vi "LET Output v1.vi"() -> ()   [LabVIEW 2010]
doc: "Cont(inuous) Acq(uire) & Chart (hw timed) demonstrates the hardware timed, non-buffered technique of data acquisition. The scan clock on the board controls acquisition timing. Acquired scans are read directly from the device's FIFO using AI Single Scan. \n\nThe acquisition is configured with no buffer, and the on-board scan clock started at the selected scan rate. In the first loop iteration, the newest (most recent) scan is read from the FIFO. In each subsequent loop iteration AI Single Scan is called to read the oldest scan from the FIFO. Then if a scan is missed because the acquisition does not keep up, an error message will be displayed, and the acquisition stopped. Each scan is plotted on the chart after it is read. \n\nA common reason to use non-buffered acquisition is that some kind of processing needs to be done for each data point. You will probably want to add more functions to the diagram to customize this VI for your application. The acquisition rate you can achieve depends on how much processing and display the VI must do. This VI calls a subVI named My Single-Scan Processing. Add whatever processing you need to this subVI, or replace it with one of your own. The data processing subVI also demonstrates how to use error clusters in your own subVIs, so they can be included in the error data flow chain.\n\nBefore running this VI, set the values of the controls on the front panel. Select Show Help Window from the Help menu to see a description of each control. If the values you select for all the controls are values you will usually use, select Make Current Values Default from the Operate menu and save the VI. Or, you may save individual control's default values by popping up on the control, selecting Data Operations, then selecting Make Current Value Default, and saving the VI."
uses:
  <instrlib>/agilent_b2900_series/Agilent B2900 Series/Public/Configure/Measurement/Configure Measurement (Current).vi
  <instrlib>/agilent_b2900_series/Agilent B2900 Series/Public/Configure/Measurement/Configure Measurement (Voltage).vi
  <vilib>/Utility/file.llb/Write To Spreadsheet File (DBL).vi
  <instrlib>/agilent_b2900_series/Agilent B2900 Series/Agilent B2900 Series.lvlib
panel:
  out "Igs array 2":dbl[][](array[numeric])
  out "Vgs array 2":dbl[][](array[numeric])
  out "Vds array 2":dbl[][](array[numeric])
  out "Corrected PD current array 2":dbl[][](array[numeric])
  out "Ids array 2":dbl[][](array[numeric])
  out "corrected PD current array":dbl[](array[numeric])
  out "Vds array":dbl[](array[numeric])
  out "Ids array":dbl[](array[numeric])
  out "Vgs array":dbl[](array[numeric])
  out "Igs array":dbl[](array[numeric])
  in  "Tab Control":T1(tab)
  in  "keithley address":string="GPIB0::20::INSTR"
  in  "agilent address":refnum<visa-resource-name>="GPIB0::23::INSTR"
  in  "Initial Vds (V)\n(100 scans/sec)":sgl caption="Initial Vds (V)" format="%.2f"
  in  "Vds step (V)":sgl=1.0 format="%.2f"
  in  "Vds delay time":sgl=10.0 caption="Vds delay time (ms)" format="%.2f"
  in  "Vds delay after first value (ms)":sgl=10.0 format="%.2f"
  in  "Final Vds(V)":sgl=60.0 format="%.2f"
  in  "light emission ON/OFF":bool=TRUE
  in  "Vgs step (V)":sgl=20.0 format="%.2f"
  in  "Final Vgs (V)":sgl=60.0 format="%.2f"
  in  "Initial Vgs (V)":sgl format="%.2f"
  in  "Vgs hold time (ms)":i32=10
  in  "Compliance Voltage (channel 2)":dbl=60.0
  in  "Compliance Current (channel 1)":dbl=0.001
  in  "Compliance Voltage (channel 1)":dbl=60.0
  in  "Compliance Current (channel 2)":dbl=0.0001
  in  "keithley compliance limit":dbl(ring)=0.025 items=["25uA"=2.5e-05, "250uA"=0.00025, "2.5mA"=0.0025, "25mA"=0.025]
  in  "Loop":bool=TRUE
  out "Current Scan":cluster{dbl[], dbl[]}(graph)
  out "Applied Vds":sgl caption="current VDS (V)" format="%.2f"
  out "Applied Vgs":sgl caption="current VDS (V)" format="%.2f"
  out "Measured Ids":dbl format="%.2e"
  out "Measured Vds":dbl
  out "corrected PD current":dbl format="%^.2e"
  out "dark PD current (A)":dbl format="%^.2e"
  out "PD current":dbl format="%^.2e"
  out "Measured Igs":dbl
  out "Measured Vgs":dbl
  out "channel 2 status":bool
  out "channel 1 status":bool
  out "Current Scan 2":cluster{dbl[], dbl[]}(graph) caption="Current Scan"
  out "half  points":sgl
  out "Vds points":sgl
  out "Vgs points":sgl
  out "?":cluster{dbl[], dbl[]}[](graph)
  out "?":cluster{dbl[], dbl[]}[](graph)
  in  "error in keithley":errorcluster
  out "keithley address out":refnum<k15>
  out "error out keithley":errorcluster
  out "error out agilent":errorcluster
  out "Agilent address out":refnum<visa-resource-name>
  # "FET output v1"
  # "Drain-Source Setting"
  # "Gate Setting"
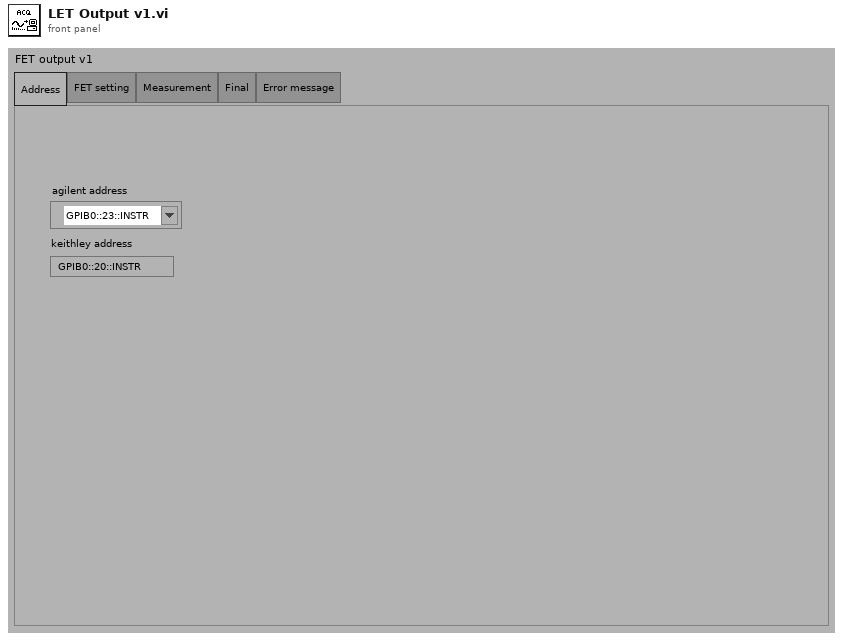
[diagram p1: front panel]
types:
  T1 = enum32{"Address", "FET setting", "Measurement", "Final", "Error message"}
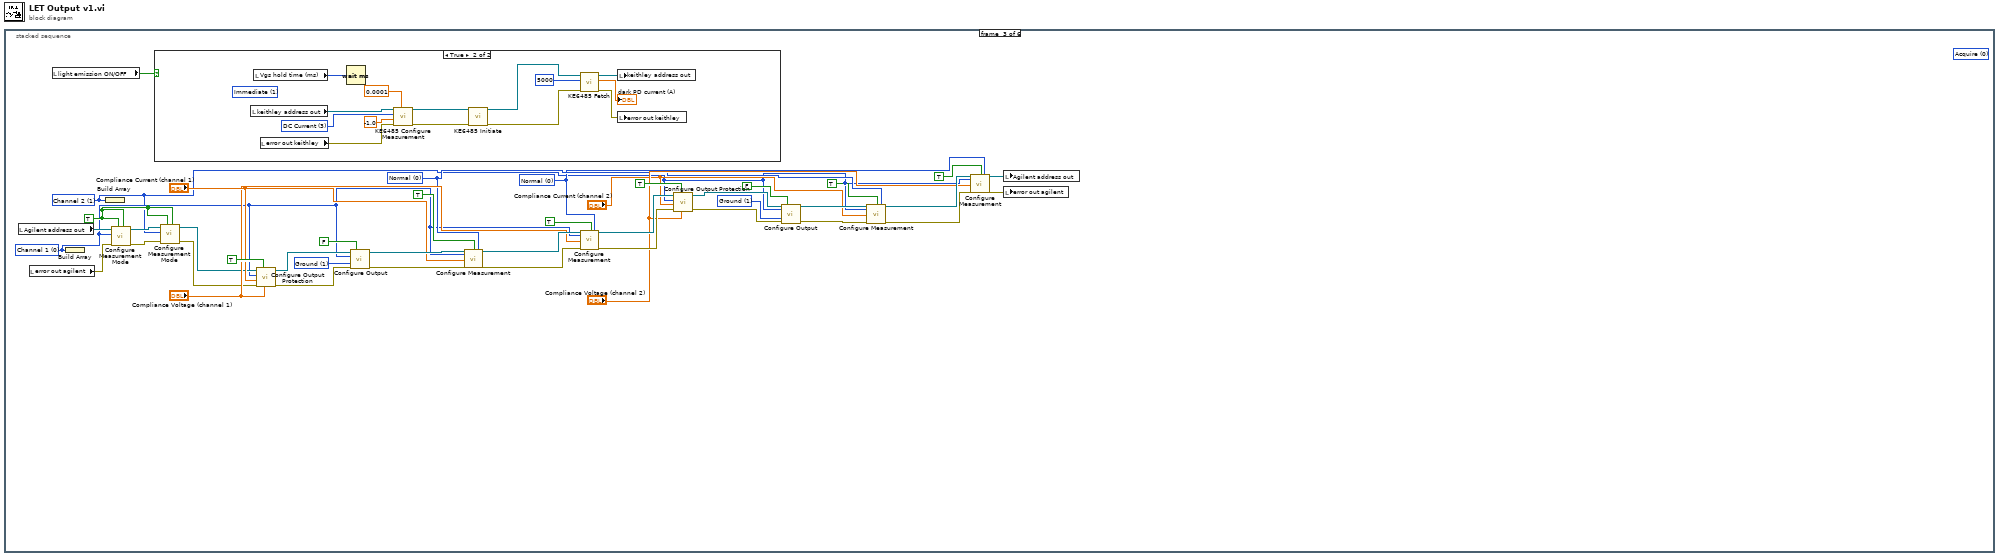
[diagram p0: block diagram]
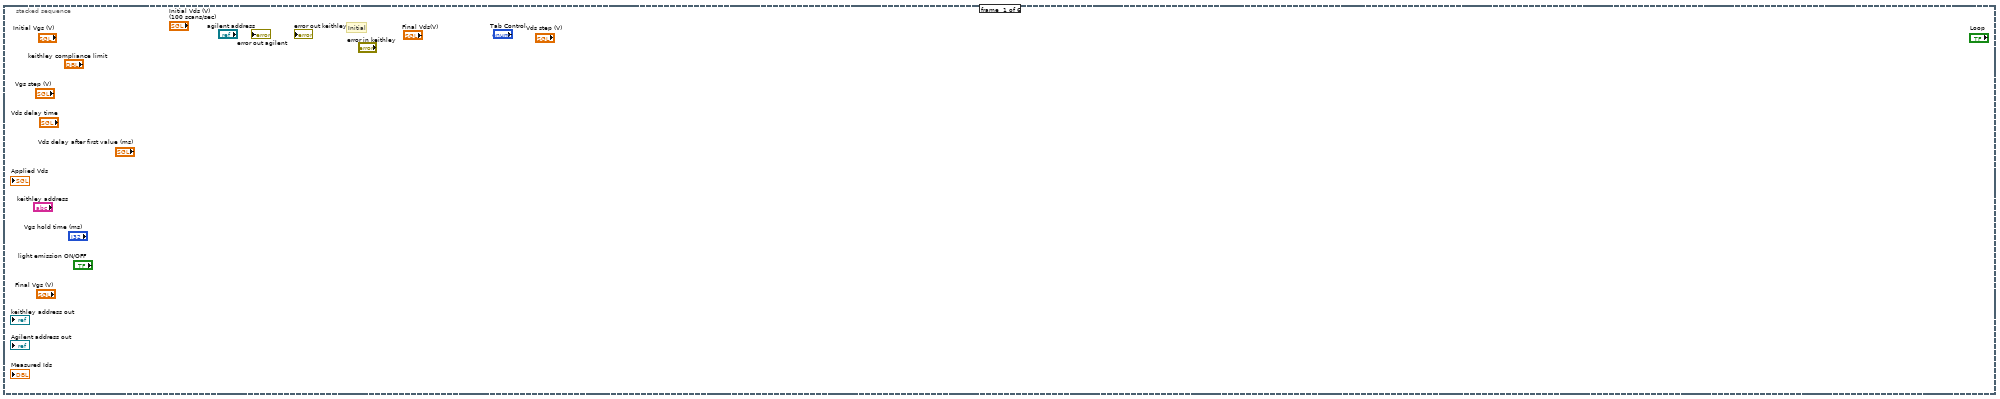
[diagram p2: hidden frame]
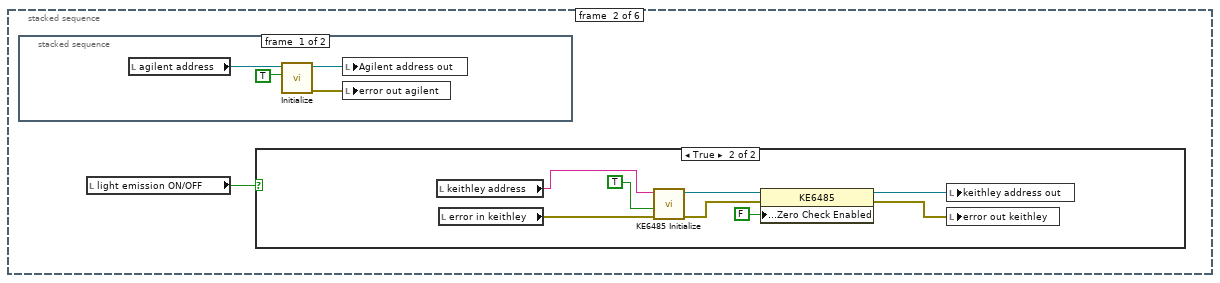
[diagram p3: hidden frame]
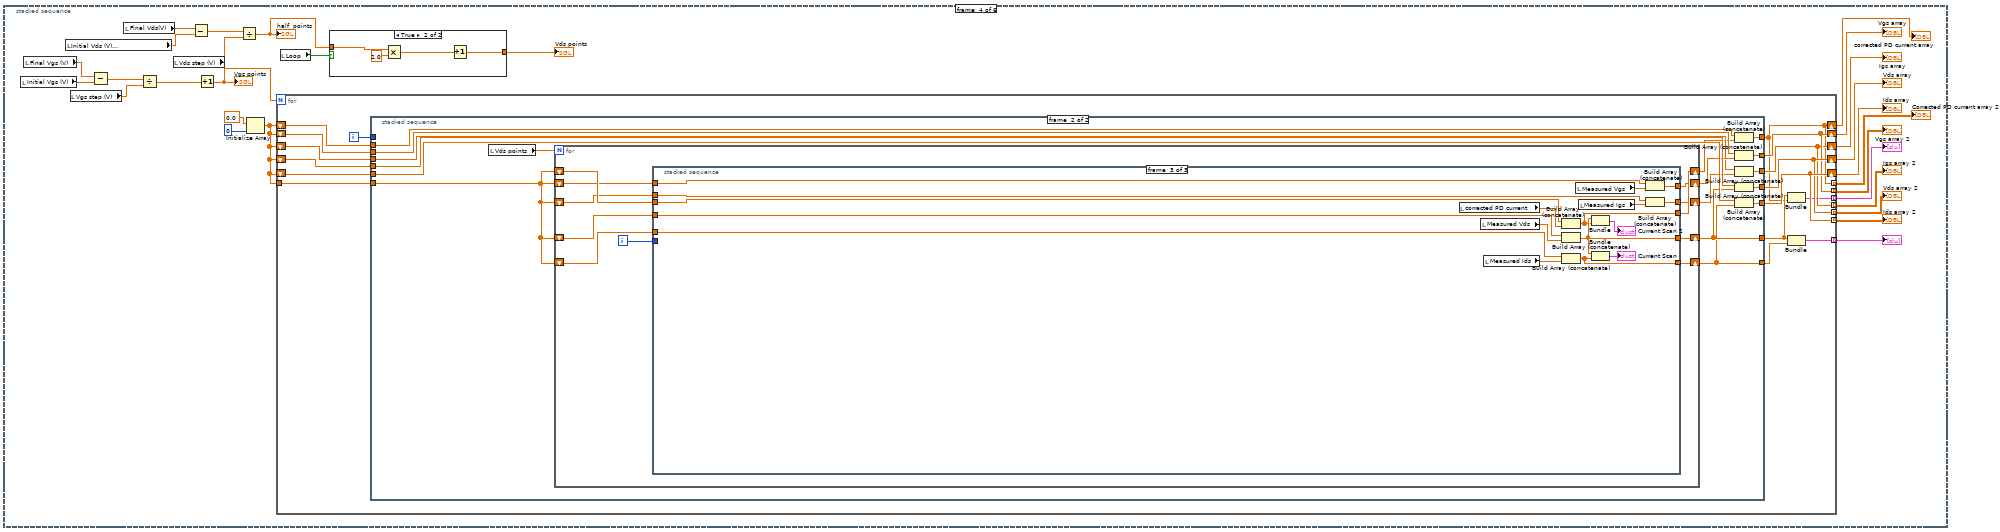
[diagram p7: hidden frame]
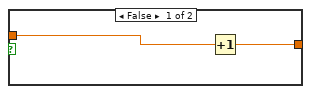
[diagram p8: hidden frame]
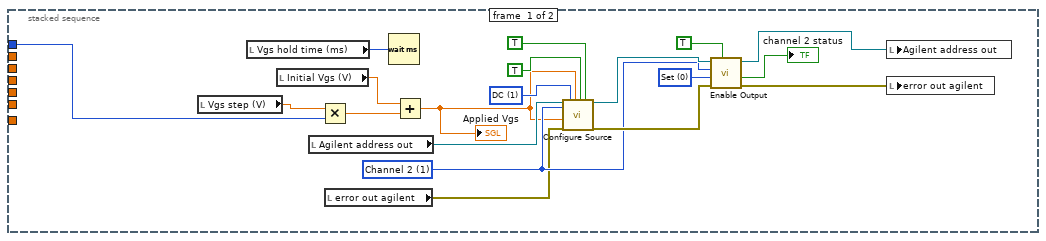
[diagram p9: hidden frame]
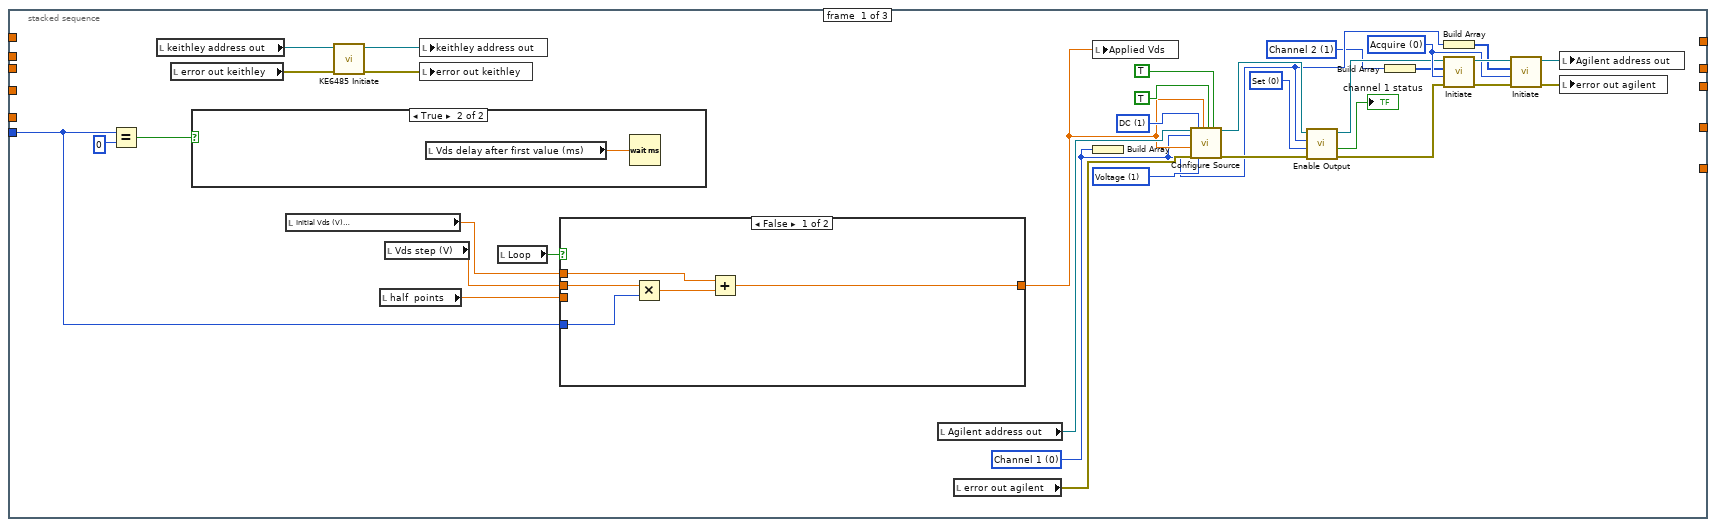
[diagram p10: hidden frame]
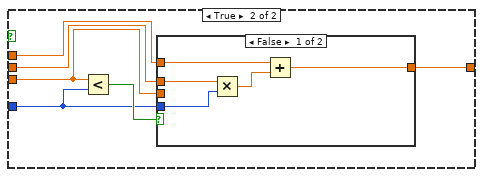
[diagram p11: hidden frame]
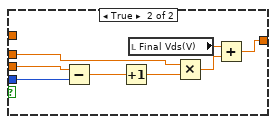
[diagram p12: hidden frame]
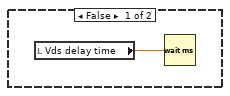
[diagram p13: hidden frame]
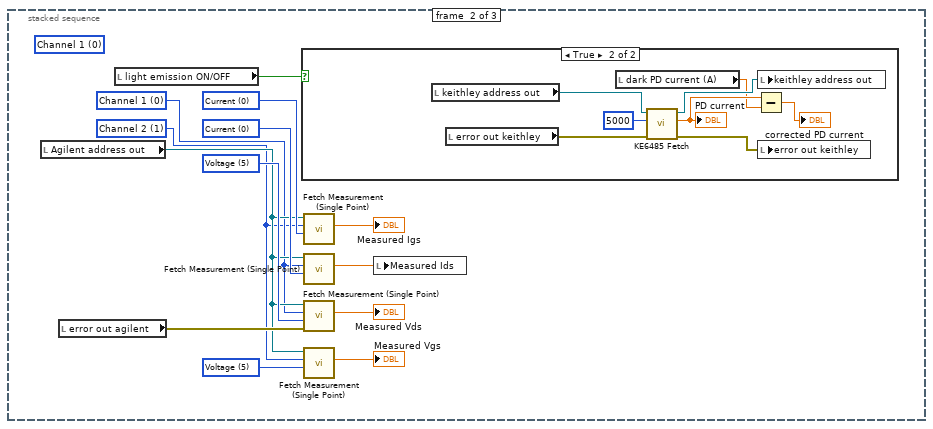
[diagram p14: hidden frame]
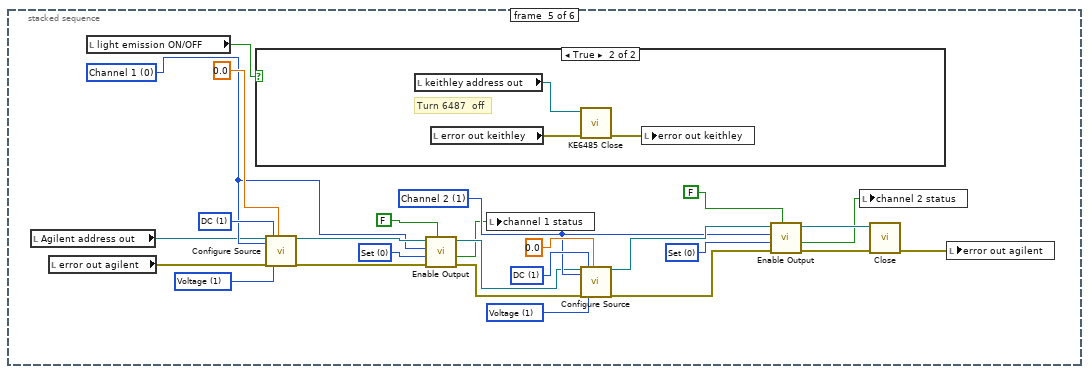
[diagram p16: hidden frame]
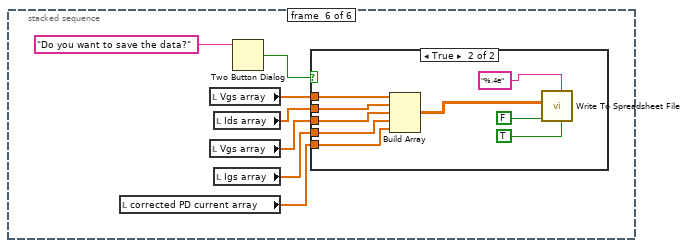
[diagram p18: hidden frame]
diagram:
  n1 = stacked-sequence {
    frame #0 {
      # "Initial"
    }
    frame #1 {
      n2 = stacked-sequence {
        frame #0 {
          n3 = local read "agilent address"() -> (w2:refnum<visa-resource-name>)
          n4 = call <instrlib>:"Initialize.vi"("ID Query (True)"=TRUE, "VISA resource name"=w2) -> ("error out"=w3:errorcluster, "VISA resource name out"=w4:refnum<visa-resource-name>)  [unwired: 8 in]
          n5 = local write "Agilent address out"(w4) -> ()
          n6 = local write "error out agilent"(w3) -> ()
        }
        frame #1 {
        }
      }
      n7 = local read "light emission ON/OFF"() -> (w1:bool)
      n8 = case shown="True" w1 {
        frame False {
        }
        frame True {
          n9 = local read "keithley address"() -> (w12:string)
          n10 = local read "error in keithley"() -> (w13:errorcluster)
          n11 = call <instrlib>:"KE6485 Initialize.vi"("error in (no error)"=w13, "reset device"=TRUE, "resource name"=w12) -> ("error out"=w10:errorcluster, "instrument handle out"=w9:refnum<k15>)  [unwired: 1 in, 6 out]
          n12 = property class="KE6485"(reference=w9, error in=w10, "System Settings:Zero Check Enabled"=FALSE) -> (reference out=w8:refnum<k15>, error out=w7:errorcluster)
          n13 = local write "keithley address out"(w8) -> ()
          n14 = local write "error out keithley"(w7) -> ()
        }
      }
    }
    frame #2 {
      (unwired) 0 items=["Acquire", "Transient", "Both"] ("Device Action (2: Both)")
      w24 = TRUE ("Enable Voltage Measurement (T: Enable)")
      w38 = 1 items=["Float", "Ground"] ("Low Terminal State (1: Ground)")
      w16 = 1 items=["Channel 1", "Channel 2"] ("Channel (0: Channel 1)")
      w26 = 0 items=["Normal", "Resolution", "Speed"] ("Current Auto Range Mode (0: Normal)")
      w48 = 1 items=["Float", "Ground"] ("Low Terminal State (1: Ground)")
      w17 = 0 items=["Channel 1", "Channel 2"] ("Channel (0: Channel 1)")
      w25 = 0 items=["Normal", "Resolution", "Speed"] ("Voltage Auto Range Mode (0: Normal)")
      n15 = local read "Agilent address out"() -> (w19:refnum<visa-resource-name>)
      n16 = local read "error out agilent"() -> (w21:errorcluster)
      n17 = local read "light emission ON/OFF"() -> (w55:bool)
      n18 = Build Array(w17) -> ()  [unwired: 1 out]
      n19 = Build Array(w16) -> ()  [unwired: 1 out]
      n20 = call <instrlib>:"Configure Measurement Mode.vi"("Enable Current Measurement (T: Enable)"=w24, "Enable Voltage Measurement (T: Enable)"=w24, "error in (no error)"=w21, "Channel (0: Channel 1)"=w17, "VISA resource name"=w19) -> ("error out"=w22:errorcluster, "VISA resource name out"=w23:refnum<visa-resource-name>)  [unwired: 5 in]
      n21 = case shown="True" w55 {
        frame False {
        }
        frame True {
          (unwired) 1 items=["Immediate"=1, "Interval"=10, "Trigger Link 1"=1001, "Trigger Link 2"=1002, "Trigger Link 3"=1003, "Trigger Link 4"=1004, "Trigger Link 5"=1005, "Trigger Link 6"=1006] ("sample trigger")
          w67 = 3 items=["DC Volts"=1, "DC Current"=3, "2 Wire Resistance"=5, "Charge"=1004] ("measurement function")
          n22 = local read "keithley address out"() -> (w62:refnum<k15>)
          n23 = local read "Vgs hold time (ms)"() -> (w69:i32)
          n24 = local read "error out keithley"() -> (w61:errorcluster)
          n25 = Wait (ms)(milliseconds to wait=w69) -> ()  [unwired: 1 out]
          n26 = call <instrlib>:"KE6485 Configure Measurement.vi"("resolution (absolute)"=0.0001, "error in (no error)"=w61, "range"=-1.0, "measurement function"=w67, "instrument handle"=w62) -> ("error out"=w58:errorcluster, "instrument handle out"=w60:refnum<k15>)  [unwired: 5 in]
          n27 = call <instrlib>:"KE6485 Initiate.vi"("error in (no error)"=w58, "instrument handle"=w60) -> ("error out"=w57:errorcluster, "instrument handle out"=w59:refnum<k15>)  [unwired: 8 in]
          n28 = call <instrlib>:"KE6485 Fetch.vi"("error in (no error)"=w57, "maximum time (ms)"=5000, "instrument handle"=w59) -> ("error out"=w64:errorcluster, "reading"=→"dark PD current (A)":dbl, "instrument handle out"=w63:refnum<k15>)  [unwired: 6 in]
          n29 = local write "keithley address out"(w63) -> ()
          n30 = local write "error out keithley"(w64) -> ()
        }
      }
      n31 = call <instrlib>:"Configure Measurement Mode.vi"("Enable Current Measurement (T: Enable)"=w24, "Enable Voltage Measurement (T: Enable)"=w24, "error in (no error)"=w22, "Channel (0: Channel 1)"=w16, "VISA resource name"=w23) -> ("error out"=w20:errorcluster, "VISA resource name out"=w18:refnum<visa-resource-name>)  [unwired: 5 in]
      n32 = call <instrlib>:"Configure Output Protection.vi"("Compliance Voltage (2 V)"="Compliance Voltage (channel 1)", "Enable Output Protection (T: Enable)"=TRUE, "error in (no error)"=w20, "Compliance Current (0.0001 A)"="Compliance Current (channel 1)", "Channel (0: Channel 1)"=w17, "VISA resource name"=w18) -> ("error out"=w50:errorcluster, "VISA resource name out"=w49:refnum<visa-resource-name>)  [unwired: 4 in]
      n33 = call <instrlib>:"Configure Output.vi"("VISA resource name"=w49, "Auto Output-Off (F: Disable)"=FALSE, "Channel (0: Channel 1)"=w17, "Low Terminal State (1: Ground)"=w48, "error in (no error)"=w50) -> ("VISA resource name out"=w46:refnum<visa-resource-name>, "error out"=w47:errorcluster)  [unwired: 9 in]
      n34 = call-poly <instrlib>:"Configure Measurement.vi"("VISA resource name"=w46, "Channel (0: Channel 1)"=w17, "Current Range (0.0001 A)"="Compliance Current (channel 1)", "error in (no error)"=w47, "Current Auto Range (T: Enable)"=TRUE, "Current Auto Range Mode (0: Normal)"=w26) -> ("VISA resource name out"=w54:refnum<visa-resource-name>, "error out"=w53:errorcluster)  [unwired: 12 in]
      n35 = call-poly <instrlib>:"Configure Measurement.vi"("VISA resource name"=w54, "Channel (0: Channel 1)"=w17, "Voltage Range (2 V)"="Compliance Voltage (channel 1)", "error in (no error)"=w53, "Voltage Auto Range (T: Enable)"=TRUE, "Voltage Auto Range Mode (0: Normal)"=w25) -> ("VISA resource name out"=w34:refnum<visa-resource-name>, "error out"=w33:errorcluster)  [unwired: 12 in]
      n36 = call <instrlib>:"Configure Output Protection.vi"("Compliance Voltage (2 V)"="Compliance Voltage (channel 2)", "Enable Output Protection (T: Enable)"=TRUE, "error in (no error)"=w33, "Compliance Current (0.0001 A)"="Compliance Current (channel 2)", "Channel (0: Channel 1)"=w16, "VISA resource name"=w34) -> ("error out"=w40:errorcluster, "VISA resource name out"=w39:refnum<visa-resource-name>)  [unwired: 4 in]
      n37 = call <instrlib>:"Configure Output.vi"("VISA resource name"=w39, "Auto Output-Off (F: Disable)"=FALSE, "Channel (0: Channel 1)"=w16, "Low Terminal State (1: Ground)"=w38, "error in (no error)"=w40) -> ("VISA resource name out"=w36:refnum<visa-resource-name>, "error out"=w37:errorcluster)  [unwired: 9 in]
      n38 = call-poly <instrlib>:"Configure Measurement.vi"("VISA resource name"=w36, "Channel (0: Channel 1)"=w16, "Current Range (0.0001 A)"="Compliance Current (channel 2)", "error in (no error)"=w37, "Current Auto Range (T: Enable)"=TRUE, "Current Auto Range Mode (0: Normal)"=w26) -> ("VISA resource name out"=w44:refnum<visa-resource-name>, "error out"=w43:errorcluster)  [unwired: 12 in]
      n39 = call-poly <instrlib>:"Configure Measurement.vi"("VISA resource name"=w44, "Channel (0: Channel 1)"=w16, "Voltage Range (2 V)"="Compliance Voltage (channel 2)", "error in (no error)"=w43, "Voltage Auto Range (T: Enable)"=TRUE, "Voltage Auto Range Mode (0: Normal)"=w25) -> ("VISA resource name out"=w15:refnum<visa-resource-name>, "error out"=w14:errorcluster)  [unwired: 12 in]
      n40 = local write "Agilent address out"(w15) -> ()
      n41 = local write "error out agilent"(w14) -> ()
    }
    frame #3 {
      n42 = local read "Initial Vgs (V)"() -> (w86:sgl)
      n43 = local read "Final Vgs (V)"() -> (w85:sgl)
      n44 = local read "Initial Vds (V)\n(100 scans/sec)"() -> (w89:sgl)
      n45 = local read "Vgs step (V)"() -> (w87:sgl)
      n46 = Subtract(x=w85, y=w86) -> (x-y=w83:sgl)
      n47 = local read "Final Vds(V)"() -> (w88:sgl)
      n48 = Divide(x=w83, y=w87) -> (x/y=w84:sgl)
      n49 = local read "Vds step (V)"() -> (w90:sgl)
      n50 = Subtract(x=w88, y=w89) -> (x-y=w97:sgl)
      n51 = Increment(x=w84) -> (x+1=w82:sgl)
      "Vgs points" <- w82
      n52 = Divide(x=w97, y=w90) -> (x/y=w79:sgl)
      "half  points" <- w79
      n53 = Initialize Array(0.0, 0) -> (w76:dbl[])
      n54 = for {
        N: w82 -> [_]
        shift-right: [w110] -> w93
        shift-left: w76 -> [w118]
        shift-right: [w111] -> w94
        shift-left: w76 -> [w117]
        shift-right: [w108] -> w92
        shift-left: w76 -> [w116]
        tunnel: [w115] -> w91 mode=indexing
        shift-right: [w107] -> w78
        shift-left: w76 -> [w114]
        shift-right: [w105] -> w77
        shift-left: w76 -> [w113]
        tunnel: w76 -> [w112]
        tunnel: [w111] -> w75 mode=indexing
        tunnel: [w105] -> w74 mode=indexing
        tunnel: [w110] -> w73 mode=indexing
        tunnel: [w108] -> w72 mode=indexing
        tunnel: [w107] -> w71 mode=indexing
        tunnel: [w104] -> w70 mode=indexing
        i -> [w119]
        n55 = stacked-sequence {
          tunnel: w119 -> [w134 _]
          tunnel: w118 -> [_ w155]
          tunnel: w117 -> [_ w154]
          tunnel: [_ w149] -> w110
          tunnel: [_ w153] -> w111
          tunnel: w116 -> [_ w151]
          tunnel: [_ w150] -> w108
          tunnel: [_ w148] -> w106
          tunnel: [_ w147] -> w109
          tunnel: w114 -> [_ w146]
          tunnel: [_ w145] -> w107
          tunnel: [_ w143] -> w105
          tunnel: w113 -> [_ w141]
          tunnel: w112 -> [_ w139]
          frame #0 {
            w127 = 0 items=["Set", "Get"] ("Operation (0: Set)")
            w128 = 1 items=["Channel 1", "Channel 2"] ("Channel (0: Channel 1)")
            w131 = 1 items=["Pulse", "DC"] ("Source Shape (1: DC)")
            n56 = local read "Vgs step (V)"() -> (w138:sgl)
            n57 = local read "Vgs hold time (ms)"() -> (w136:i32)
            n58 = local read "Initial Vgs (V)"() -> (w137:sgl)
            n59 = local read "Agilent address out"() -> (w124:refnum<visa-resource-name>)
            n60 = Multiply(x=w138, y=w134) -> (x*y=w135:sgl)
            n61 = local read "error out agilent"() -> (w123:errorcluster)
            n62 = Wait (ms)(milliseconds to wait=w136) -> ()  [unwired: 1 out]
            n63 = Add(x=w137, y=w135) -> (x+y=w120:sgl)
            "Applied Vgs" <- w120
            n64 = call <instrlib>:"Configure Source.vi"("VISA resource name"=w124, "Channel (0: Channel 1)"=w128, "Source Range (2)"=w120, "error in (no error)"=w123, "Source Shape (1: DC)"=w131, "Output Level (0)"=w120, "Source Auto Range (T: Enable)"=TRUE, "Enable Continuous Output (T: Enable)"=TRUE) -> ("VISA resource name out"=w133:refnum<visa-resource-name>, "error out"=w132:errorcluster)  [unwired: 10 in]
            n65 = call <instrlib>:"Enable Output.vi"("Enable Output (T: Enable)"=TRUE, "error in (no error)"=w132, "Operation (0: Set)"=w127, "Channel (0: Channel 1)"=w128, "VISA resource name"=w133) -> ("error out"=w122:errorcluster, "Output Enabled?"=→"channel 2 status":bool, "VISA resource name out"=w121:refnum<visa-resource-name>)  [unwired: 4 in]
            n66 = local write "Agilent address out"(w121) -> ()
            n67 = local write "error out agilent"(w122) -> ()
          }
          frame #1 {
            n68 = local read "Vds points"() -> (w140:sgl)
            n69 = for {
              N: w140 -> [_]
              shift-right: [w157] -> w147
              shift-left: w139 -> [w156]
              shift-right: [w159] -> w148
              shift-left: w139 -> [w158]
              shift-right: [w163] -> w152
              shift-left: w139 -> [w162]
              shift-right: [w161] -> w144
              shift-left: w139 -> [w160]
              shift-right: [w164] -> w142
              shift-left: w139 -> [w165]
              i -> [w166]
              n70 = stacked-sequence {
                tunnel: w166 -> [w186 _ _]
                tunnel: w165 -> [_ _ w262]
                tunnel: [_ _ w247] -> w164
                tunnel: [_ _ w260] -> w163
                tunnel: w162 -> [_ _ w259]
                tunnel: [_ _ w257] -> w161
                tunnel: w160 -> [_ _ w256]
                tunnel: [_ _ w248] -> w159
                tunnel: w158 -> [_ _ w253]
                tunnel: [_ _ w250] -> w157
                tunnel: w156 -> [_ _ w251]
                frame #0 {
                  w179 = 0 items=["Acquire", "Transient", "Both"] ("Device Action (2: Both)")
                  w171 = 1 items=["Channel 1", "Channel 2"] ("Channel (0: Channel 1)")
                  w188 = 1 items=["Current", "Voltage"] ("Source Mode (1: Voltage)")
                  w191 = 1 items=["Pulse", "DC"] ("Source Shape (1: DC)")
                  w172 = 0 items=["Channel 1", "Channel 2"] ("Channel (0: Channel 1)")
                  w195 = 0 items=["Set", "Get"] ("Operation (0: Set)")
                  n71 = Equal?(x=w186, y=0) -> (x = y?=w198:bool)
                  n72 = local read "keithley address out"() -> (w168:refnum<k15>)
                  n73 = local read "error out keithley"() -> (w167:errorcluster)
                  n74 = case shown="True" w198 {
                    frame False {
                      n75 = local read "Vds delay time"() -> (w224:sgl)
                      n76 = Wait (ms)(milliseconds to wait=w224) -> ()  [unwired: 1 out]
                    }
                    frame True {
                      n77 = local read "Vds delay after first value (ms)"() -> (w225:sgl)
                      n78 = Wait (ms)(milliseconds to wait=w225) -> ()  [unwired: 1 out]
                    }
                  }
                  n79 = local read "Initial Vds (V)\n(100 scans/sec)"() -> (w187:sgl)
                  n80 = call <instrlib>:"KE6485 Initiate.vi"("error in (no error)"=w167, "instrument handle"=w168) -> ("error out"=w170:errorcluster, "instrument handle out"=w169:refnum<k15>)  [unwired: 8 in]
                  n81 = local read "half  points"() -> (w183:sgl)
                  n82 = local read "Vds step (V)"() -> (w185:sgl)
                  n83 = local write "keithley address out"(w169) -> ()
                  n84 = local write "error out keithley"(w170) -> ()
                  n85 = local read "Loop"() -> (w184:bool)
                  n86 = case shown="False" w184 {
                    tunnel: [w203 w209] -> w182
                    tunnel: w186 -> [w202 w206]
                    tunnel: w187 -> [w201 w208]
                    tunnel: w185 -> [w200 w207]
                    tunnel: w183 -> [_ w205]
                    frame False {
                      n87 = Multiply(x=w200, y=w202) -> (x*y=w204:sgl)
                      n88 = Add(x=w201, y=w204) -> (x+y=w203:sgl)
                    }
                    frame True {
                      n89 = Less?(x=w205, y=w206) -> (x < y?=w210:bool)
                      n90 = case shown="False" w210 {
                        tunnel: [w214 w223] -> w209
                        tunnel: w208 -> [w213 _]
                        tunnel: w206 -> [w212 w220]
                        tunnel: w207 -> [w211 w221]
                        tunnel: w205 -> [_ w219]
                        frame False {
                          n91 = Multiply(x=w211, y=w212) -> (x*y=w215:sgl)
                          n92 = Add(x=w213, y=w215) -> (x+y=w214:sgl)
                        }
                        frame True {
                          n93 = Subtract(x=w219, y=w220) -> (x-y=w217:sgl)
                          n94 = Increment(x=w217) -> (x+1=w216:sgl)
                          n95 = local read "Final Vds(V)"() -> (w218:sgl)
                          n96 = Multiply(x=w221, y=w216) -> (x*y=w222:sgl)
                          n97 = Add(x=w218, y=w222) -> (x+y=w223:sgl)
                        }
                      }
                    }
                  }
                  n98 = local read "Agilent address out"() -> (w193:refnum<visa-resource-name>)
                  n99 = local read "error out agilent"() -> (w192:errorcluster)
                  n100 = local write "Applied Vds"(w182) -> ()
                  n101 = Build Array(w172) -> ()  [unwired: 1 out]
                  n102 = call <instrlib>:"Configure Source.vi"("VISA resource name"=w193, "Channel (0: Channel 1)"=w172, "Source Range (2)"=w182, "error in (no error)"=w192, "Source Shape (1: DC)"=w191, "Source Mode (1: Voltage)"=w188, "Output Level (0)"=w182, "Source Auto Range (T: Enable)"=TRUE, "Enable Continuous Output (T: Enable)"=TRUE) -> ("VISA resource name out"=w197:refnum<visa-resource-name>, "error out"=w196:errorcluster)  [unwired: 9 in]
                  n103 = call <instrlib>:"Enable Output.vi"("error in (no error)"=w196, "Operation (0: Set)"=w195, "Channel (0: Channel 1)"=w172, "VISA resource name"=w197) -> ("error out"=w175:errorcluster, "Output Enabled?"=→"channel 1 status":bool, "VISA resource name out"=w176:refnum<visa-resource-name>)  [unwired: 5 in]
                  n104 = Build Array(w171) -> (w178:i32[])
                  n105 = Build Array(w172) -> (w177:i32[])
                  n106 = call <instrlib>:"Initiate.vi"("error in (no error)"=w175, "Device Action (2: Both)"=w179, "Channel List ({Channel1})"=w178, "VISA resource name"=w176) -> ("error out"=w181:errorcluster, "VISA resource name out"=w180:refnum<visa-resource-name>)  [unwired: 6 in]
                  n107 = call <instrlib>:"Initiate.vi"("error in (no error)"=w181, "Device Action (2: Both)"=w179, "Channel List ({Channel1})"=w177, "VISA resource name"=w180) -> ("error out"=w174:errorcluster, "VISA resource name out"=w173:refnum<visa-resource-name>)  [unwired: 6 in]
                  n108 = local write "Agilent address out"(w173) -> ()
                  n109 = local write "error out agilent"(w174) -> ()
                }
                frame #1 {
                  w227 = 1 items=["Channel 1", "Channel 2"] ("Channel (0: Channel 1)")
                  w228 = 0 items=["Channel 1", "Channel 2"] ("Channel (0: Channel 1)")
                  w233 = 0 items=["Current", "Resistance", "Source Output Setting", "Status", "Time", "Voltage"] ("Data Mode (5: Voltage)")
                  w234 = 5 items=["Current", "Resistance", "Source Output Setting", "Status", "Time", "Voltage"] ("Data Mode (5: Voltage)")
                  w236 = 0 items=["Current", "Resistance", "Source Output Setting", "Status", "Time", "Voltage"] ("Data Mode (5: Voltage)")
                  (unwired) 0 items=["Channel 1", "Channel 2"] ("Channel (0: Channel 1)")
                  w238 = 5 items=["Current", "Resistance", "Source Output Setting", "Status", "Time", "Voltage"] ("Data Mode (5: Voltage)")
                  n110 = local read "Agilent address out"() -> (w229:refnum<visa-resource-name>)
                  n111 = local read "error out agilent"() -> (w230:errorcluster)
                  n112 = local read "light emission ON/OFF"() -> (w226:bool)
                  n113 = case shown="True" w226 {
                    frame False {
                    }
                    frame True {
                      n114 = local read "keithley address out"() -> (w240:refnum<k15>)
                      n115 = local read "error out keithley"() -> (w239:errorcluster)
                      n116 = local read "dark PD current (A)"() -> (w241:dbl)
                      n117 = call <instrlib>:"KE6485 Fetch.vi"("error in (no error)"=w239, "maximum time (ms)"=5000, "instrument handle"=w240) -> ("error out"=w245:errorcluster, "reading"=w242:dbl, "instrument handle out"=w244:refnum<k15>)  [unwired: 6 in]
                      "PD current" <- w242
                      n118 = Subtract(x=w242, y=w241) -> (x-y=→"corrected PD current":dbl)
                      n119 = local write "keithley address out"(w244) -> ()
                      n120 = local write "error out keithley"(w245) -> ()
                    }
                  }
                  n121 = call <instrlib>:"Fetch Measurement (Single Point).vi"("Data Mode (5: Voltage)"=w233, "Channel (0: Channel 1)"=w227, "VISA resource name"=w229) -> ("Measurement"=→"Measured Igs":dbl)  [unwired: 6 in, 2 out]
                  n122 = call <instrlib>:"Fetch Measurement (Single Point).vi"("Data Mode (5: Voltage)"=w236, "Channel (0: Channel 1)"=w228, "VISA resource name"=w229) -> ("Measurement"=w235:dbl)  [unwired: 6 in, 2 out]
                  n123 = call <instrlib>:"Fetch Measurement (Single Point).vi"("error in (no error)"=w230, "Data Mode (5: Voltage)"=w238, "Channel (0: Channel 1)"=w228, "VISA resource name"=w229) -> ("Measurement"=→"Measured Vds":dbl)  [unwired: 5 in, 2 out]
                  n124 = call <instrlib>:"Fetch Measurement (Single Point).vi"("Data Mode (5: Voltage)"=w234, "Channel (0: Channel 1)"=w227, "VISA resource name"=w229) -> ("Measurement"=→"Measured Vgs":dbl)  [unwired: 6 in, 2 out]
                  n125 = local write "Measured Ids"(w235) -> ()
                }
                frame #2 {
                  n126 = local read "corrected PD current"() -> (w263:dbl)
                  n127 = local read "Measured Vds"() -> (w254:dbl)
                  n128 = local read "Measured Ids"() -> (w252:dbl)
                  n129 = Build Array (concatenate)(w262, w263) -> (w247:dbl[])
                  n130 = Build Array (concatenate)(w253, w254) -> (w248:dbl[])
                  n131 = Build Array (concatenate)(w251, w252) -> (w250:dbl[])
                  n132 = local read "Measured Vgs"() -> (w261:dbl)
                  n133 = local read "Measured Igs"() -> (w258:dbl)
                  n134 = Bundle(w248, w247) -> (→"Current Scan 2":cluster{dbl[], dbl[]})  [unwired: 1 out]
                  n135 = Bundle(w248, w250) -> (→"Current Scan":cluster{dbl[], dbl[]})  [unwired: 1 out]
                  n136 = Build Array (concatenate)(w259, w261) -> (w260:dbl[])
                  n137 = Build Array (concatenate)(w256, w258) -> (w257:dbl[])
                }
              }
            }
            n138 = Build Array (concatenate)(w141, w142) -> (w143:dbl[])
            n139 = Build Array (concatenate)(w151, w152) -> (w150:dbl[])
            n140 = Build Array (concatenate)(w146, w144) -> (w145:dbl[])
            n141 = Build Array (concatenate)(w155, w148) -> (w149:dbl[])
            n142 = Build Array (concatenate)(w154, w147) -> (w153:dbl[])
          }
        }
        n143 = Bundle(w106, w105) -> (w104:cluster{dbl[], dbl[]})  [unwired: 1 out]
        n144 = Bundle(w106, w109) -> (w115:cluster{dbl[], dbl[]})  [unwired: 1 out]
      }
      "?" <- w91
      "Igs array" <- w78
      "Vgs array" <- w92
      "Ids array" <- w94
      "Vds array" <- w93
      "corrected PD current array" <- w77
      "Ids array 2" <- w75
      "Corrected PD current array 2" <- w74
      "Vds array 2" <- w73
      "Vgs array 2" <- w72
      "Igs array 2" <- w71
      "?" <- w70
      n145 = local read "Loop"() -> (w80:bool)
      n146 = case shown="True" w80 {
        tunnel: w79 -> [w99 w103]
        tunnel: [w98 w101] -> w81
        frame False {
          n147 = Increment(x=w99) -> (x+1=w98:sgl)
        }
        frame True {
          n148 = Multiply(x=w103, y=sgl 2.0) -> (x*y=w100:sgl)
          n149 = Increment(x=w100) -> (x+1=w101:sgl)
        }
      }
      "Vds points" <- w81
    }
    frame #4 {
      w274 = 0 items=["Set", "Get"] ("Operation (0: Set)")
      w276 = 1 items=["Current", "Voltage"] ("Source Mode (1: Voltage)")
      w273 = 1 items=["Channel 1", "Channel 2"] ("Channel (0: Channel 1)")
      w277 = 1 items=["Pulse", "DC"] ("Source Shape (1: DC)")
      w282 = 0 items=["Set", "Get"] ("Operation (0: Set)")
      w284 = 1 items=["Current", "Voltage"] ("Source Mode (1: Voltage)")
      w281 = 0 items=["Channel 1", "Channel 2"] ("Channel (0: Channel 1)")
      w285 = 1 items=["Pulse", "DC"] ("Source Shape (1: DC)")
      n150 = local read "Agilent address out"() -> (w265:refnum<visa-resource-name>)
      n151 = local read "error out agilent"() -> (w264:errorcluster)
      n152 = local read "light emission ON/OFF"() -> (w289:bool)
      n153 = case shown="True" w289 {
        frame False {
        }
        frame True {
          # "Turn 6487  off"
          n154 = local read "keithley address out"() -> (w291:refnum<k15>)
          n155 = local read "error out keithley"() -> (w290:errorcluster)
          n156 = call <instrlib>:"KE6485 Close.vi"("error in (no error)"=w290, "instrument handle"=w291) -> ("error out"=w292:errorcluster)  [unwired: 9 out]
          n157 = local write "error out keithley"(w292) -> ()
        }
      }
      n158 = call <instrlib>:"Configure Source.vi"("VISA resource name"=w265, "Channel (0: Channel 1)"=w281, "error in (no error)"=w264, "Source Shape (1: DC)"=w285, "Source Mode (1: Voltage)"=w284, "Output Level (0)"=0.0) -> ("VISA resource name out"=w287:refnum<visa-resource-name>, "error out"=w283:errorcluster)  [unwired: 12 in]
      n159 = call <instrlib>:"Enable Output.vi"("Enable Output (T: Enable)"=FALSE, "error in (no error)"=w283, "Operation (0: Set)"=w282, "Channel (0: Channel 1)"=w281, "VISA resource name"=w287) -> ("error out"=w271:errorcluster, "Output Enabled?"=w267:bool, "VISA resource name out"=w272:refnum<visa-resource-name>)  [unwired: 4 in]
      n160 = local write "channel 1 status"(w267) -> ()
      n161 = call <instrlib>:"Configure Source.vi"("VISA resource name"=w272, "Channel (0: Channel 1)"=w273, "error in (no error)"=w271, "Source Shape (1: DC)"=w277, "Source Mode (1: Voltage)"=w276, "Output Level (0)"=0.0) -> ("VISA resource name out"=w279:refnum<visa-resource-name>, "error out"=w275:errorcluster)  [unwired: 12 in]
      n162 = call <instrlib>:"Enable Output.vi"("Enable Output (T: Enable)"=FALSE, "error in (no error)"=w275, "Operation (0: Set)"=w274, "Channel (0: Channel 1)"=w273, "VISA resource name"=w279) -> ("error out"=w270:errorcluster, "Output Enabled?"=w268:bool, "VISA resource name out"=w269:refnum<visa-resource-name>)  [unwired: 4 in]
      n163 = local write "channel 2 status"(w268) -> ()
      n164 = call <instrlib>:"Close.vi"("error in (no error)"=w270, "VISA resource name"=w269) -> ("error out"=w266:errorcluster)  [unwired: 9 in]
      n165 = local write "error out agilent"(w266) -> ()
    }
    frame #5 {
      n166 = local read "corrected PD current array"() -> (w294:dbl[])
      n167 = local read "Vgs array"() -> (w293:dbl[])
      n168 = local read "Vgs array"() -> (w296:dbl[])
      n169 = local read "Ids array"() -> (w297:dbl[])
      n170 = local read "Igs array"() -> (w295:dbl[])
      n171 = Two Button Dialog(message="Do you want to save the data?") -> (T button?=w298:bool)  [unwired: 2 out]
      n172 = case shown="True" w298 {
        tunnel: w296 -> [_ w305]
        tunnel: w297 -> [_ w304]
        tunnel: w295 -> [_ w301]
        tunnel: w294 -> [_ w300]
        tunnel: w293 -> [_ w303]
        frame False {
        }
        frame True {
          n173 = Build Array(w303, w304, w305, w301, w300) -> (w302:dbl[][])
          n174 = call-poly <vilib>:"Write To Spreadsheet File.vi"("transpose? (no:F)"=TRUE, "format (%.3f)"="%.4e", "append to file? (new file:F)"=FALSE, "2D data"=w302) -> ()  [unwired: 4 in, 1 out]
        }
      }
    }
  }
